vi "LINX - Servo.vi"() -> ()   [LabVIEW 2011, in "LVH-LINX.lvlib"]
uses:
  vi.lib/LabVIEW Hacker/LINX/LVH-LINX.lvlib
  vi.lib/LabVIEW Hacker/LINX/Public/Sensors/Motion/Servo/Servo.lvlib
panel:
  in  "Stop Button":bool
  in  "Pulse Width (uS)":u16[](array[numeric])
  in  "Serial Port":refnum<visa-resource-name>="N/A"
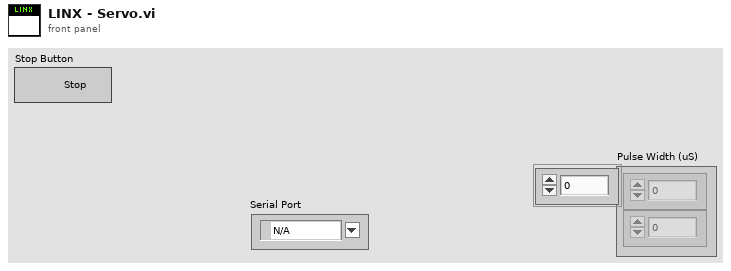
[diagram p1: front panel]
types:
  T1 = typedef "LVH-LINX.lvlib/LINX Ref.ctl" = cluster{"Platform":T2, "Interface":T3, "LINX Device Config":T4}
  T2 = typedef "LVH-LINX.lvlib/Platform.ctl" = enum16{"LINX", "myRIO"}
  T3 = typedef "LVH-LINX.lvlib/Interface.ctl" = enum16{"Serial", "TCP"}
  T4 = typedef "LVH-LINX.lvlib/Device.lvlib/LINX Device Config.ctl" = cluster{"Interface":T3, "COM Port":refnum<visa-resource-name>, "TCP Configuration":T5, "Device Family":u8, "Device ID":u8, "Device Name":string, "TCP Ref":refnum<k5>, "Channels":T6}
  T5 = typedef "LVH-LINX.lvlib/Device.lvlib/TCP Config.ctl" = cluster{"IP Address":string, "Port":u16}
  T6 = typedef "LVH-LINX.lvlib/Channels.ctl" = cluster{"DI":u8[], "DO":u8[], "AI":u8[], "AO":u8[], "PWM":u8[], "QE":u8[], "UART":u8[], "I2C 2":u8[], "SPI":u8[], "CAN":u8[], "Servo":u8[], "AI Ref (V)":dbl, "AO Ref (V)":dbl, "AO Resolution (Bits)":u8}
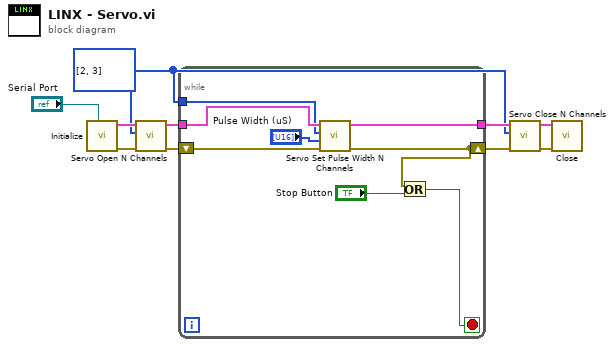
[diagram p0: block diagram]
diagram:
  w1 = u8[] [2, 3] ("Servo Channels")
  n1 = call "Initialize.vi"("Serial Port"="Serial Port") -> ("Error Out"=w10:errorcluster, "LINX Ref"=w3:T1)  [unwired: 8 in, 1 out]
  n2 = call "Servo Open N Channels.vi"("Error In"=w10, "Servo Channels"=w1, "LINX Resource"=w3) -> ("Error Out"=w9:errorcluster, "LINX Resource"=w4:T1)  [unwired: 7 in]
  n3 = while {
    tunnel: [w17] -> w5
    tunnel: w4 -> [w16]
    shift-right: [w12] -> w8
    shift-left: w9 -> [w18]
    tunnel: w1 -> [w15]
    stop <- w13 stop-if-true
    n4 = call "Servo Set Pulse Width N Channels.vi"("Error In"=w18, "Pulse Widths (uS)"="Pulse Width (uS)", "Servo Channels"=w15, "LINX Resource"=w16) -> ("Error Out"=w12:errorcluster, "LINX Resource"=w17:T1)  [unwired: 6 in]
    n5 = Or(x=w12, y="Stop Button") -> (x .or. y?=w13:bool)
  }
  n6 = call "Servo Close N Channels.vi"("Error In"=w8, "Servo Channels"=w1, "LINX Resource"=w5) -> ("Error Out"=w7:errorcluster, "LINX Resource"=w6:T1)  [unwired: 7 in]
  n7 = call "Close.vi"("Error In"=w7, "LINX Resource"=w6) -> ()  [unwired: 8 in, 2 out]
